vi "Scrape Screenpops.vi"(8 "error in":errorcluster, 9 "UI":refnum<queue>, 11 "SR number list in":i32[](array[numeric])) -> (0 "error out":errorcluster, 1 "sr notes array out":T1[][](array[typedef]) {"Note Date" format="%<%x >T"}, 3 "sr clusters out":T2[](array[typedef]) {"Creation Date" format="%<%x>T"; "Last Updated" format="%<%x>T"})   [LabVIEW 2018]
uses:
  Type Defs/SR Cluster.ctl
  Type Defs/SR Status.ctl
  Type Defs/SR Note Cluster.ctl
  Support/Message Queue/Message Cluster.ctl
  Support/Message Queue/Enqueue Message (Single).vi
  <vilib>/httpClient/LabVIEWHTTPClient.lvlib
  Support/Message Queue/Message Queue.lvlib
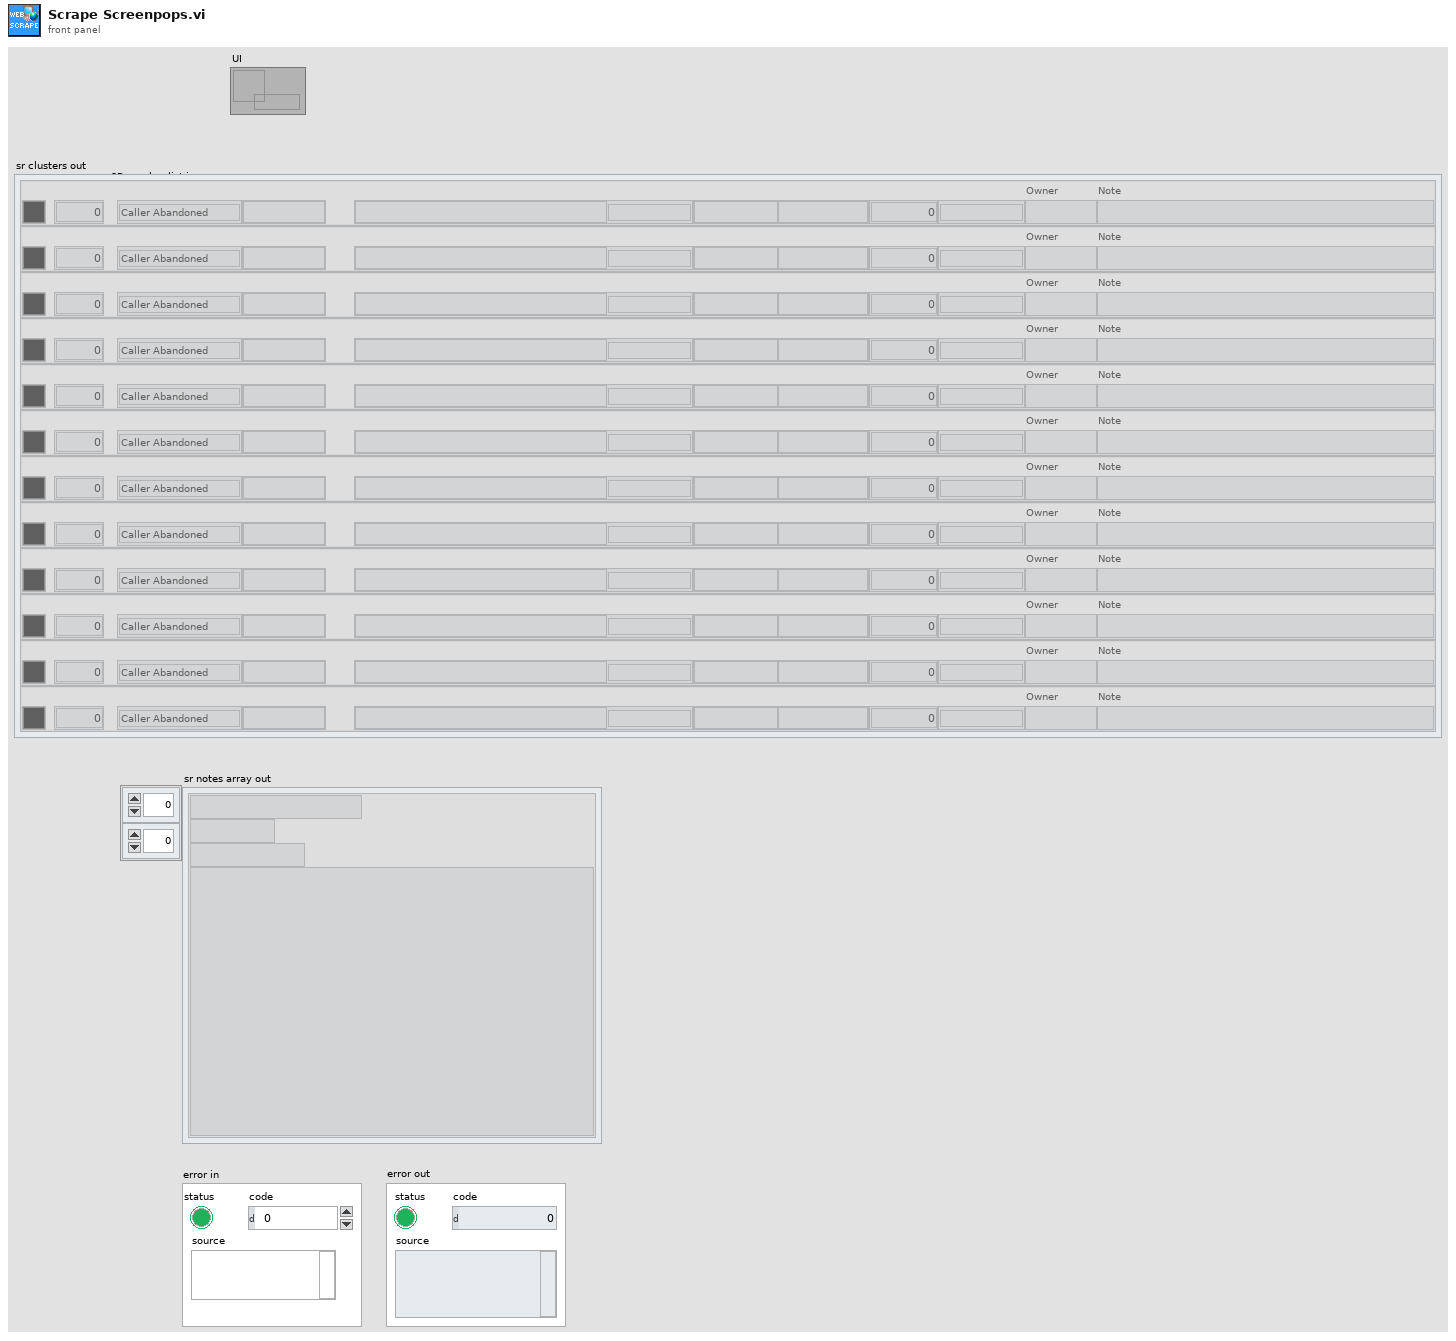
[diagram p1: front panel]
types:
  T1 = typedef "SR Note Cluster.ctl" = cluster{"Note Type":string, "Note Date":timestamp, "AE":string, "Note Text":string}
  T2 = typedef "SR Cluster.ctl" = cluster{"Color":u32, "SR Number":i32, "SR Status":T3, "Name":string, "Summary":string, "Last Updated":timestamp, "SR Type":string, "Service Level":string, "Days Open":dbl, "Creation Date":timestamp, "Owner":string, "Note":string}
  T3 = typedef "SR Status.ctl" = enum16{"Caller Abandoned", "Created in Error", "Expired", "Forum Resolved AE", "Forum Resolved Customer", "IN WORK", "IN WORK Collab with AES", "IN WORK Collab with PSE", "IN WORK Collab with SE", "IN WORK Customer Added Note", "IN WORK Escalation", "IN WORK Wait on Customer", "Open", "Potentially Resolved", "Presumed Resolved", "RMA Approved for Return", "RMA Closed", "RMA Closed - DOA", "RMA In Progress", "RMA Open", "RMA Waiting on Customer", "Resolved", "Passed Off"}
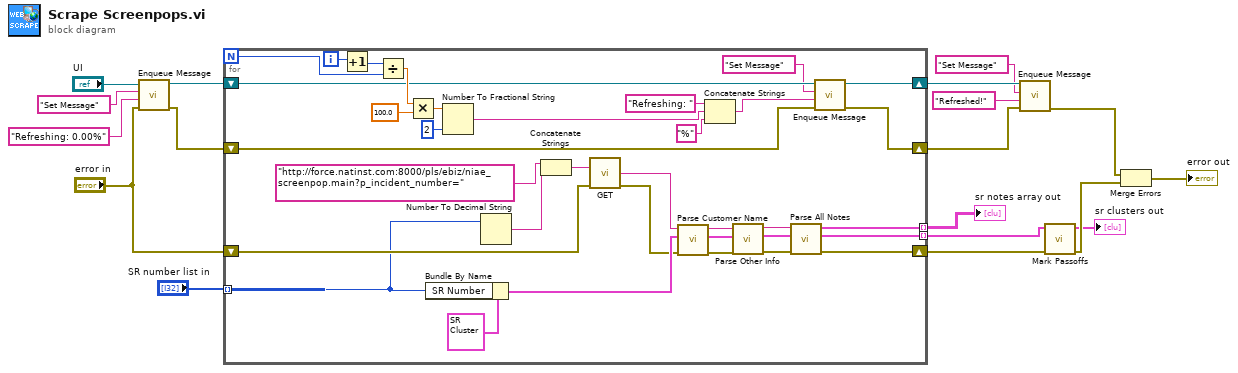
[diagram p0: block diagram]
diagram:
  n1 = call-poly "Enqueue Message.vi"("error in (no error)"="error in", "Message Data"="Refreshing: 0.00%" ("Message"), "Message"="Set Message", "Message Queue"="UI") -> ("error out"=w8:errorcluster, "dup Message Queue"=w13:refnum<queue>)  [unwired: 6 in]
  n2 = for {
    N -> [w28]
    tunnel: "SR number list in" -> [w47] mode=indexing
    tunnel: [w48] -> w1 mode=indexing
    tunnel: [w46] -> w17 mode=indexing
    shift-right: [w20] -> w6
    shift-left: "error in" -> [w52]
    shift-right: [w29] -> w12
    shift-left: w13 -> [w37]
    shift-right: [w21] -> w7
    shift-left: w8 -> [w22]
    i -> [w27]
    n3 = Increment(x=w27) -> (x+1=w26:i32)
    n4 = Divide(x=w26, y=w28) -> (x/y=w38:dbl)
    n5 = Multiply(x=w38, y=100.0) -> (x*y=w32:dbl)
    n6 = Bundle By Name(cluster=T2 {"Color"=0, "SR Number"=0, "SR Status"=enum."Caller Abandoned", "Name"="", "Summary"="", "Last Updated"=timestamp(0 s since 1904-01-01), "SR Type"="", "Service Level"="", "Days Open"=0.0, "Creation Date"=timestamp(0 s since 1904-01-01), "Owner"="", "Note"=""} ("SR Cluster"), "SR Number"=w47) -> (w44:T2)
    n7 = Number To Fractional String(number=w32, precision (6)=i16 2) -> (F-format string=w30:string)  [unwired: 2 in]
    n8 = Number To Decimal String(number=w47) -> (decimal integer string=w51:string)  [unwired: 1 in]
    n9 = Concatenate Strings("http://force.natinst.com:8000/pls/ebiz/niae_screenpop.main?p_incident_number=" ("string"), w51) -> (w50:string)
    n10 = call <vilib>:"GET.vi"("url"=w50, "error in (no error)"=w52) -> ("body"=w45:string, "error out"=w24:errorcluster)  [unwired: 10 in, 2 out]
    n11 = call "Parse Customer Name.vi"("error in"=w24, "SR Cluster in"=w44, "HTML text in"=w45) -> ("error out"=w23:errorcluster, "SR Cluster out"=w43:T2, "remaining string out"=w42:string)  [unwired: 6 in]
    n12 = Concatenate Strings("Refreshing: " ("string"), w30, "%" ("string")) -> (w34:string)
    n13 = call "Parse Other Info.vi"("error in (no error)"=w23, "SR Cluster in"=w43, "remaining string in"=w42) -> ("error out"=w39:errorcluster, "SR Cluster out"=w40:T2, "result string"=w41:string)  [unwired: 6 in]
    n14 = call "Parse All Notes.vi"("error in (no error)"=w39, "SR Cluster in"=w40, "result string"=w41) -> ("error out"=w20:errorcluster, "SR Cluster out"=w48:T2, "Array"=w46:T1[])  [unwired: 6 in]
    n15 = call-poly "Enqueue Message.vi"("error in (no error)"=w22, "Message Data"=w34, "Message"="Set Message", "Message Queue"=w37) -> ("error out"=w21:errorcluster, "dup Message Queue"=w29:refnum<queue>)  [unwired: 6 in]
  }
  "sr notes array out" <- w17
  n16 = call-poly "Enqueue Message.vi"("error in (no error)"=w7, "Message Data"="Refreshed!" ("string"), "Message"="Set Message", "Message Queue"=w12) -> ("error out"=w3:errorcluster)  [unwired: 6 in, 1 out]
  n17 = call "Mark Passoffs.vi"("error in"=w6, "Array in"=w1) -> ("error out"=w4:errorcluster, "Array out"=→"sr clusters out":T2[])  [unwired: 8 in]
  n18 = Merge Errors(w3, w4) -> (→"error out":errorcluster)
